vi "Library Explain Error.vi"(0 "explanation prefix (none)":string, 9 "skip levels (0)":i32, 11 "error in (no error)":errorcluster) -> (15 "explained error":errorcluster)   [LabVIEW 2013]
doc: "This VI assists with constructing and explaining errors. The error is prefixed with explanation text and appended with any call chain.\n\nThis VI examines the input error to see if it is already explained, in which case the error is either passed out unmodified or a further explanation, if provided, is prefixed. Consequently, there is no problem with using this VI at multiple points along an error chain. Use this VI to construct new errors, when there is some additional information that further clarifies the error, or when the error is about to be displayed and there could be some as yet unexplained error code. Depending on the values of the inputs, this VI has several modes of operation.\n\nWhen no explanation is wired, and the input is left unwired or a \"no error\" value is passed, the output error will be a duplicate of the input \"no error\".\n\nWhen the input error is left unwired or a \"no error\" value is passed yet the explanation is wired, a new error is constructed. To do so, the source is assumed to be the calling VI (unless skip levels is used) and a source string is constructed from the call chain. To this the provided explanation prefix is prepended. The resulting explanation is set as the source string of the output error cluster. Also, the magic error code (9876) is set to indicate that the source holds an explanation.\n\nWhen an explanation prefix is wired, and an error is input that is already is explained (has the magic error code), the explanation prefix is prepended to the source string as a further elaboration.\n\nWhen no explanation prefix is wired and an error is input that is already explained (has the magic error code), it will be passed out unmodified.\n\nWhen an error is input that is not explained, it will be looked up in the error code database and the retrieved explanation will be appended to its source (which LabVIEW should have set to some call chain and optional node). Next, any provided prefix is prepended and the whole is set as the source of the output error which will also have the magic error code."
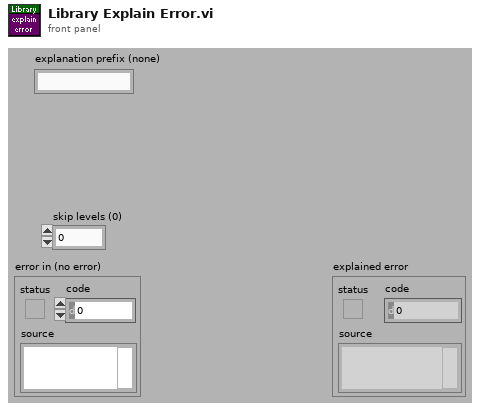
[diagram p1: front panel]
types:
  T1 = cluster{bool, "magic error code":i32, "explanation prefix (none)":string}
  T2 = cluster{bool, "magic error code":i32, "source":string}
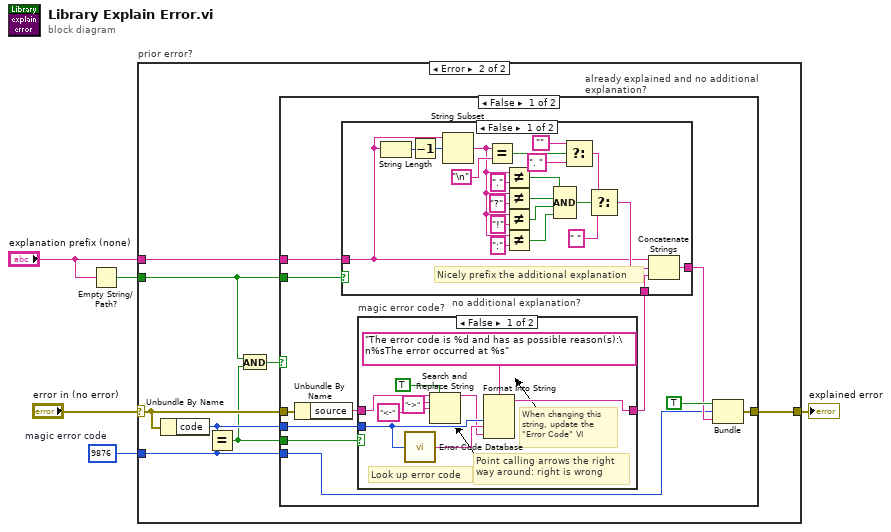
[diagram p0: block diagram]
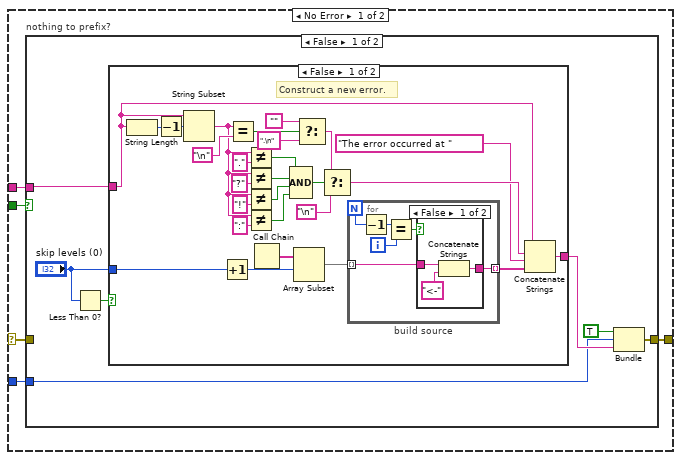
[diagram p2: hidden frame]
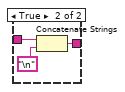
[diagram p3: hidden frame]
diagram:
  w1 = 9876  # magic error code
  n1 = Empty String/Path?(string/path="explanation prefix (none)") -> (empty?=w2:bool)
  n2 = case "prior error?" shown="Error" "error in (no error)" {
    selector: "error in (no error)" -> [w10 w65]
    tunnel: "explanation prefix (none)" -> [w6 w61]
    tunnel: [w9 w62] -> w3
    tunnel: w2 -> [w8 w60]
    tunnel: w1 -> [w7 w59]
    frame No Error {
      n3 = case "nothing to prefix?" shown="False" w8 {
        tunnel: w10 -> [_ w58]
        tunnel: [w14 w58] -> w9
        tunnel: w7 -> [w15 _]
        tunnel: w6 -> [w17 _]
        frame False {
          n4 = Less Than 0?(x="skip levels (0)") -> (x < 0?=w12:bool)
          n5 = case shown="False" w12 {
            tunnel: w17 -> [w20 w57]
            tunnel: "skip levels (0)" -> [w31 _]
            tunnel: [w18 w57] -> w16
            frame False {
              # "Construct a new error."
              n6 = String Length(string=w20) -> (length=w38:i32)
              n7 = Decrement(x=w38) -> (x-1=w39:i32)
              n8 = String Subset(string=w20, offset (0)=w39) -> (substring=w22:string)  [unwired: 1 in]
              n9 = Increment(x=w31) -> (x+1=w34:i32)
              n10 = Equal?(x=w22, y="\n") -> (x = y?=w40:bool)
              n11 = Not Equal?(x=w22, y=".") -> (x != y?=w25:bool)
              n12 = Not Equal?(x=w22, y="?") -> (x != y?=w27:bool)
              n13 = Not Equal?(x=w22, y="!") -> (x != y?=w26:bool)
              n14 = Not Equal?(x=w22, y=":") -> (x != y?=w21:bool)
              n15 = Call Chain() -> (call chain=w33:string[])
              n16 = Compound Arithmetic op=AND(w25, w27, w26, w21) -> (w24:bool)
              n17 = Array Subset(array=w33, index=w34) -> (w32:string[])  [unwired: 1 in]
              n18 = Select(t="", s=w40, f=".\n") -> (s? t:f=w42:string)
              n19 = Select(t=w42, s=w24, f="\n") -> (s? t:f=w43:string)
              n20 = for "build source" {
                N -> [w50]
                tunnel: w32 -> [w46] mode=indexing
                tunnel: [w45] -> w19 mode=indexing
                i -> [w48]
                n21 = Decrement(x=w50) -> (x-1=w49:i32)
                n22 = Equal?(x=w49, y=w48) -> (x = y?=w47:bool)
                n23 = case shown="False" w47 {
                  tunnel: w46 -> [w52 w56]
                  tunnel: [w51 w54] -> w45
                  frame False {
                    n24 = Concatenate Strings(w52, "<-") -> (w51:string)
                  }
                  frame True {
                    n25 = Concatenate Strings(w56, "\n") -> (w54:string)
                  }
                }
              }
              n26 = Concatenate Strings(w20, w43, "The error occurred at ", w19) -> (w18:string)
            }
            frame True {
              # "Reconstruct an old explained error (temporarily stored as a string)."
            }
          }
          n27 = Bundle(TRUE, "magic error code"=w15, "explanation prefix (none)"=w16) -> (w14:T1)  [unwired: 1 in]
        }
        frame True {
        }
      }
    }
    frame Error {
      n28 = Unbundle By Name(w65) -> ("code"=w66:i32)
      n29 = Equal?(x=w66, y=w59) -> (x = y?=w64:bool)
      n30 = And(x=w60, y=w64) -> (x .and. y?=w63:bool)
      n31 = case "already explained and no additional explanation?" shown="False" w63 {
        tunnel: w66 -> [w77 _]
        tunnel: w65 -> [w75 w111]
        tunnel: w64 -> [w76 _]
        tunnel: [w67 w111] -> w62
        tunnel: w61 -> [w73 _]
        tunnel: w60 -> [w72 _]
        tunnel: w59 -> [w68 _]
        frame False {
          n32 = Unbundle By Name(w75) -> ("source"=w74:string)
          n33 = case "magic error code?" shown="False" w76 {
            tunnel: [w108 w110] -> w71
            tunnel: w77 -> [w103 _]
            tunnel: w74 -> [w106 w110]
            frame False {
              # "Point calling arrows the right\nway around: right is wrong"
              # "When changing this\nstring, update the\n\"Error Code\" VI"
              # "Look up error code"
              n34 = call <vilib>:"Error Code Database.vi"("Error Code"=w103) -> ("Error Text"=w102:string)
              n35 = Search and Replace String(replace all?=TRUE ("replace all? (F)"), input string=w106, search string="->", replace string="<-" ("replace string (\"\")")) -> (result string=w101:string)  [unwired: 4 in, 3 out]
              n36 = Format Into String(format string="The error code is %d and has as possible reason(s):\n%sThe error occurred at %s", w103, w102, w101) -> (resulting string=w108:string)  [unwired: 2 in, 1 out]
            }
            frame True {
              # "This should already be a proper explanation"
            }
          }
          n37 = case "no additional explanation?" shown="False" w72 {
            tunnel: w73 -> [w89 _]
            tunnel: w71 -> [w88 w100]
            tunnel: [w87 w100] -> w69
            frame False {
              # "Nicely prefix the additional explanation"
              n38 = String Length(string=w89) -> (length=w93:i32)
              n39 = Decrement(x=w93) -> (x-1=w94:i32)
              n40 = String Subset(string=w89, offset (0)=w94) -> (substring=w79:string)  [unwired: 1 in]
              n41 = Equal?(x=w79, y="\n") -> (x = y?=w95:bool)
              n42 = Not Equal?(x=w79, y=".") -> (x != y?=w82:bool)
              n43 = Not Equal?(x=w79, y="?") -> (x != y?=w84:bool)
              n44 = Not Equal?(x=w79, y="!") -> (x != y?=w83:bool)
              n45 = Not Equal?(x=w79, y=":") -> (x != y?=w78:bool)
              n46 = Compound Arithmetic op=AND(w82, w84, w83, w78) -> (w81:bool)
              n47 = Select(t="", s=w95, f=". ") -> (s? t:f=w98:string)
              n48 = Select(t=w98, s=w81, f=" ") -> (s? t:f=w90:string)
              n49 = Concatenate Strings(w89, w90, w88) -> (w87:string)
            }
            frame True {
            }
          }
          n50 = Bundle(TRUE, "magic error code"=w68, "source"=w69) -> (w67:T2)  [unwired: 1 in]
        }
        frame True {
        }
      }
    }
  }
  "explained error" <- w3
